vi "Ensure Default CellStyle.vi"(8 "error in":errorcluster, 11 "SpreadsheetDoc in":refnum<k24>) -> (0 "error out":errorcluster, 3 "SpreadsheetDoc out":refnum<k24>)   [LabVIEW 2021, in "Open Xml.lvlib"]
uses:
  Open Xml.lvlib
  D:/git/Open-Xml-LabVIEW/dll/DocumentFormat.OpenXml.dll
  dll/DocumentFormat.OpenXml.dll
  D:/git/Open-Xml-LabVIEW/dll/DocumentFormat.OpenXml.Framework.dll
  dll/DocumentFormat.OpenXml.Framework.dll
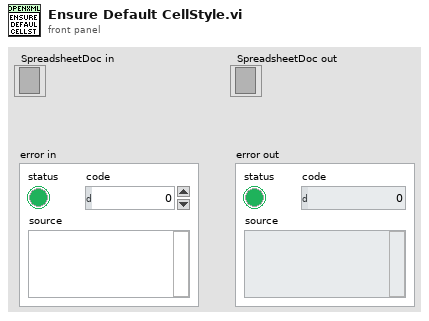
[diagram p1: front panel]
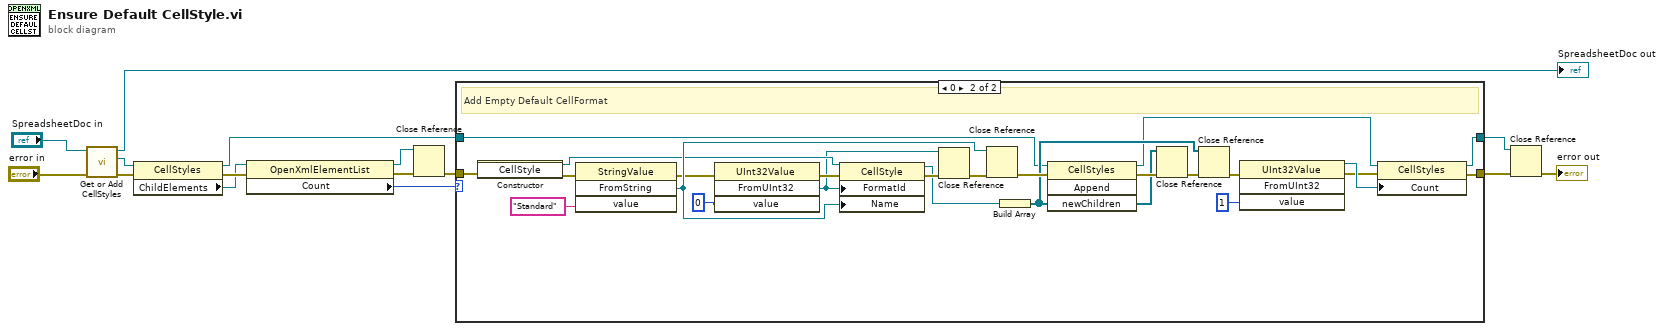
[diagram p0: block diagram]
diagram:
  n1 = call "Get or Add CellStyles.vi"("error in"="error in", "SpreadsheetDoc in"="SpreadsheetDoc in") -> ("error out"=w12:errorcluster, "CellStyles"=w11:refnum<k24>, "SpreadsheetDoc out"=→"SpreadsheetDoc out":refnum<k24>)  [unwired: 7 in]
  n2 = property class="CellStyles"(reference=w11, error in=w12) -> (reference out=w4:refnum<k24>, error out=w10:errorcluster, "ChildElements"=w7:refnum<k24>)
  n3 = property class="OpenXmlElementList"(reference=w7, error in=w10) -> (reference out=w6:refnum<k24>, error out=w8:errorcluster, "Count"=w9:i32)
  n4 = Close Reference(reference=w6, error in (no error)=w8) -> (error out=w5:errorcluster)
  n5 = case shown="0" w9 {
    tunnel: w5 -> [w17 w37]
    tunnel: [w17 w25] -> w15
    tunnel: w4 -> [w16 w26]
    tunnel: [w16 w23] -> w1
    frame Default {
      # "Default"
    }
    frame 0 {
      # "Add Empty Default CellFormat"
      n6 = constructor class="CellStyle"(error in=w37) -> (reference out=w36:refnum<k24>, error out=w35:errorcluster)  [unwired: 2 in, 1 out]
      n7 = invoke class="StringValue" method="FromString"(error in=w35, "value"="Standard") -> (error out=w34:errorcluster, "FromString"=w40:refnum<k24>)  [unwired: 2 in, 2 out]
      n8 = invoke class="UInt32Value" method="FromUInt32"(error in=w34, "value"=u32 0) -> (error out=w33:errorcluster, "FromUInt32"=w31:refnum<k24>)  [unwired: 2 in, 2 out]
      n9 = property class="CellStyle"(reference=w36, error in=w33, "FormatId"=w31, "Name"=w40) -> (reference out=w38:refnum<k24>, error out=w39:errorcluster)
      n10 = Close Reference(reference=w31, error in (no error)=w39) -> (error out=w32:errorcluster)
      n11 = Close Reference(reference=w40, error in (no error)=w32) -> (error out=w41:errorcluster)
      n12 = Build Array(w38) -> (w27:refnum<k24>[])
      n13 = invoke class="CellStyles" method="Append"(reference=w26, error in=w41, "newChildren"=w27) -> (reference out=w24:refnum<k24>, error out=w30:errorcluster, "newChildren"=w29:refnum<k24>[])  [unwired: 1 in, 1 out]
      n14 = Close Reference(reference=w29, error in (no error)=w30) -> (error out=w28:errorcluster)
      n15 = Close Reference(reference=w27, error in (no error)=w28) -> (error out=w20:errorcluster)
      n16 = invoke class="UInt32Value" method="FromUInt32"(error in=w20, "value"=u32 1) -> (reference out=w22:refnum<k24>, error out=w19:errorcluster)  [unwired: 2 in, 2 out]
      n17 = property class="CellStyles"(reference=w24, error in=w19, "Count"=w22) -> (reference out=w23:refnum<k24>, error out=w25:errorcluster)
    }
  }
  n18 = Close Reference(reference=w1, error in (no error)=w15) -> (error out=→"error out":errorcluster)
